vi "2DGaussianWithRotationFit000.vi"() -> ()   [LabVIEW 2009]
uses:
  <vilib>/gmath/NumericalOptimization/Nonlinear Curve Fit LM.vi
  <vilib>/gmath/NI_Gmath.lvlib
  <vilib>/Analysis/NI_AALBase.lvlib
panel:
  out "number of function calls":i32
  in  "stop":bool
  in  "Simulation":dbl[](array[slide])=[97.19626168224299, 146.41744548286604, 94.70404984423675, 22.429906542056074, 38.006230529595015, 127.10280373831775] caption="Amplitude\n\n\nX-Position\n\n\nY-Position\n\n\nWidth A\n\n\nWidth B\n\n\nAngle" scale=0.0..200.0
  in  "Fit!":bool
  out "Parameters":dbl[][](array[numeric]) caption="Auto Guess                  Actual              Best Fit           Difference" format="%.4f"
  in  "Noise":dbl=10.0
  out "error out":errorcluster
  out "Best Fit":dbl[][](graph)
  out "Data":dbl[][](graph)
  # "(1) Simulate desired surface by\nchanging parameters and noise\n(2) Press fit and wait a while"
  # "Widths are currently defined as\n2*sigma for code simplicity."
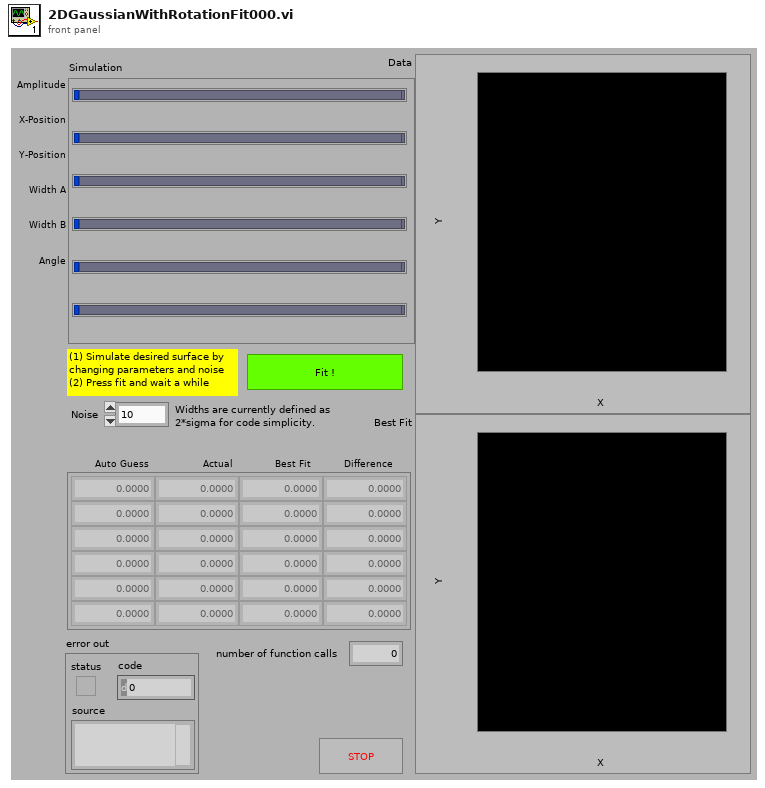
[diagram p1: front panel]
types:
  T1 = typedef "LVBoundsTypeDef.ctl" = cluster{"Width":u32, "Height":u32}
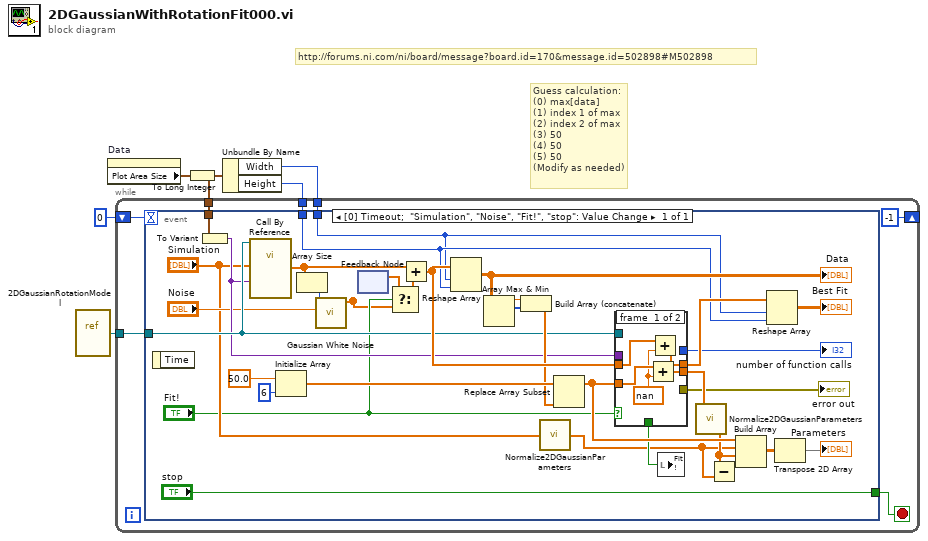
[diagram p0: block diagram]
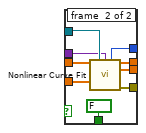
[diagram p2: hidden frame]
diagram:
  # "http://forums.ni.com/ni/board/message?board.id=170&message.id=502898#M502898"
  # "Guess calculation:\n(0) max[data]\n(1) index 1 of max\n(2) index 2 of max\n(3) 50\n(4) 50\n(5) 50\n(Modify as needed)"
  n1 = vi-ref "2DGaussianRotationModel.vi"() -> (w6:refnum<vi>)
  n2 = property on="Data" class="IntGraph (strict)"() -> ("Plot Area Size"=w5:T1)  [unwired: 2 in, 2 out]
  n3 = To Long Integer(number=w5) -> (32bit integer=w1:cluster{"Width":i32, "Height":i32})
  n4 = Unbundle By Name(w1) -> ("Width"=w3:i32, "Height"=w2:i32)
  n5 = while {
    tunnel: w6 -> [w13]
    tunnel: w1 -> [w12]
    shift-right: [-1] -> _
    shift-left: 0 -> [w9]
    tunnel: w3 -> [w8]
    tunnel: w2 -> [w7]
    stop <- w11 stop-if-true
    n6 = event shown="[0] Timeout;  \"Simulation\", \"Noise\", \"Fit!\", \"stop\": Value Change" {
      selector: _ -> [_]
      dyn-events: _ -> [_]
      timeout: w9 -> [_]
      tunnel: w13 -> [w29]
      tunnel: w12 -> [w41]
      tunnel: ["stop"] -> w11
      tunnel: w8 -> [w18]
      tunnel: w7 -> [w24]
      event [0] Timeout;  "Simulation", "Noise", "Fit!", "stop": Value Change {
        n7 = event-data() -> ()  [unwired: 1 in, 1 out]
        n8 = To Variant(anything=w41) -> (Variant=w27:variant)
        n9 = call-by-ref "?"(reference=w29, "data"=w27, "a"="Simulation") -> ("f(X,a)"=w28:dbl[])  [unwired: 3 in, 4 out]
        n10 = Initialize Array(50.0 ("element"), 6 ("dimension size")) -> (w37:dbl[])
        n11 = Array Size(array=w28) -> (size(s)=w45:i32)
        n12 = call <vilib>:"Gaussian White Noise.vi"("standard deviation"="Noise", "samples"=w45) -> ("Gaussian noise pattern"=w21:dbl[])  [unwired: 8 in, 1 out]
        n13 = feedback #1() -> (w20:dbl[])  [unwired: 1 in]
        n14 = Select(t=w20, s="Fit!", f=w21) -> (s? t:f=w23:dbl[])
        n15 = Add(x=w28, y=w23) -> (x+y=w44:dbl[])
        n16 = Reshape Array(w44, w18, w24) -> (w42:dbl[][])
        "Data" <- w42
        n17 = Array Max & Min(array=w42) -> (max value=w35:dbl, max index (indices)=w40:i32[])  [unwired: 2 out]
        n18 = Build Array (concatenate)(w35, w40) -> (w36:dbl[])
        n19 = call "Normalize2DGaussianParameters.vi"("best fit parameters IN"="Simulation") -> ("best fit parameters OUT"=w14:dbl[])
        n20 = Replace Array Subset(array=w37, new element=w36) -> (w34:dbl[])  [unwired: 1 in]
        n21 = case shown="True" "Fit!" {
          tunnel: [w49 w61] -> w47
          tunnel: [_ w60] -> w17
          tunnel: w29 -> [_ w59]
          tunnel: w27 -> [_ w58]
          tunnel: w44 -> [w52 w57]
          tunnel: [w50 w56] -> w43
          tunnel: w34 -> [w51 w55]
          tunnel: [_ w54] -> w19
          tunnel: [_ FALSE] -> w16
          frame #0 {
            w48 = nan ("element")
            n22 = Add(x=w51, y=w48) -> (x+y=w50:dbl[])
            n23 = Add(x=w52, y=w48) -> (x+y=w49:dbl[])
          }
          frame #1 {
            n24 = call-poly <vilib>:"Nonlinear Curve Fit.vi"("Y"=w57, "f(x,a)"=w59, "data"=w58, "initial parameters"=w55) -> ("number of function calls"=w54:i32, "best nonlinear fit"=w61:dbl[], "best fit parameters"=w56:dbl[], "error out"=w60:errorcluster)  [unwired: 6 in, 2 out]
          }
        }
        "error out" <- w17
        "number of function calls" <- w19
        n25 = local write "Fit!"(w16) -> ()
        n26 = call "Normalize2DGaussianParameters.vi"("best fit parameters IN"=w43) -> ("best fit parameters OUT"=w32:dbl[])
        n27 = Subtract(x=w32, y=w14) -> (x-y=w33:dbl[])
        n28 = Build Array(w34, w14, w32, w33) -> (w31:dbl[][])
        n29 = Reshape Array(w47, w18, w24) -> (→"Best Fit":dbl[][])
        n30 = Transpose 2D Array(2D array=w31) -> (transposed array=→"Parameters":dbl[][])
      }
    }
  }
